vi "toString.vi"(8 "error in (no error)":errorcluster, 11 "Pizza in":refnum<class "Pizza.lvclass">) -> (0 "error out":errorcluster, 2 "String":string, 3 "Pizza out":refnum<class "Pizza.lvclass">)   [LabVIEW 2020, in "FactoryMethod.lvlib" / "PizzaFactoryMethod.lvlib" / "Pizza.lvclass"]
uses:
  Pizza.lvclass
  Pizza.lvclass/Pizza.ctl
  Private/Property/name/Read name.vi
  Private/Property/dough/Read dough.vi
  Private/Property/sauce/Read sauce.vi
  Private/Property/toppings/Read toppings.vi
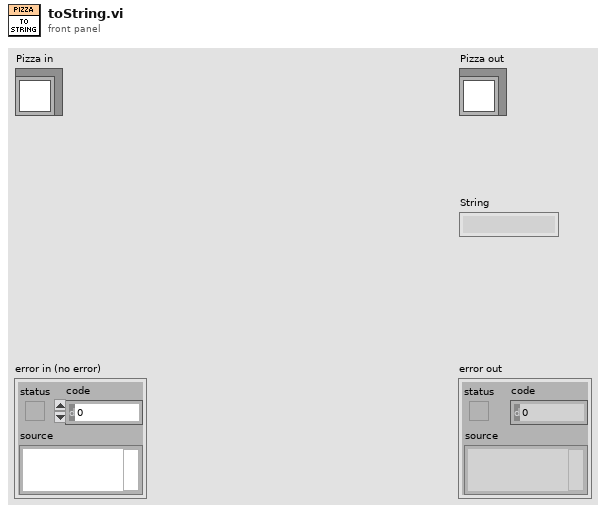
[diagram p1: front panel]
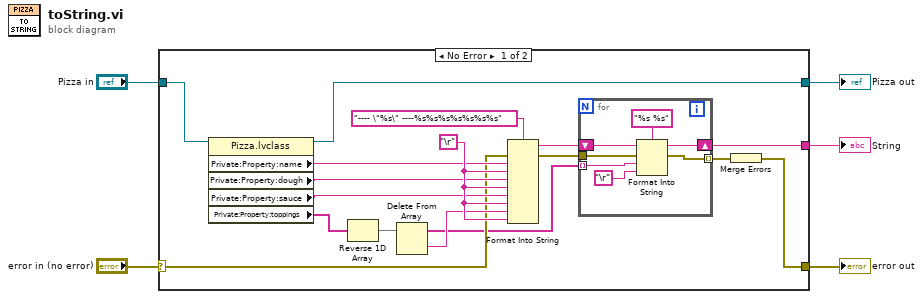
[diagram p0: block diagram]
diagram:
  n1 = case shown="No Error" "error in (no error)" {
    selector: "error in (no error)" -> [w12 w31]
    tunnel: [w21 w31] -> w4
    tunnel: [w8 w30] -> w2
    tunnel: "Pizza in" -> [w20 w30]
    tunnel: [w9 _] -> w1
    frame No Error {
      w18 = "\r"
      n2 = property class="Pizza.lvclass"(reference=w20) -> (reference out=w8:refnum<class "Pizza.lvclass">, "Private:Property:name"=w17:string, "Private:Property:dough"=w16:string, "Private:Property:sauce"=w15:string, "Private:Property:toppings"=w7:string[])  [unwired: 1 in, 1 out]
      n3 = Reverse 1D Array(array=w7) -> (reversed array=w14:string[])
      n4 = Delete From Array(array=w14) -> (deleted portion=w13:string, array with subset deleted=w6:string[])  [unwired: 2 in]
      n5 = Format Into String(format string="---- \"%s\" ----%s%s%s%s%s%s%s" ("initial string"), error in=w12, w17, w18, w16, w18, w15, w18, w13, w18) -> (resulting string=w10:string, error out=w11:errorcluster)  [unwired: 1 in]
      n6 = for {
        tunnel: w6 -> [w29] mode=indexing
        shift-right: [w28] -> w9
        shift-left: w10 -> [w27]
        tunnel: w11 -> [w26]
        tunnel: [w25] -> w22 mode=indexing
        n7 = Format Into String(format string="%s %s", initial string=w27, error in=w26, w29, "\r") -> (resulting string=w28:string, error out=w25:errorcluster)
      }
      n8 = Merge Errors(w22) -> (w21:errorcluster)
    }
    frame Error {
    }
  }
  "error out" <- w4
  "Pizza out" <- w2
  "String" <- w1
